vi "ReadFFLoop.vi"(0 "blocktrigger":u8, 1 "btrig_ch":u8, 2 "ExtTrig":u8, 3 "cam_sel":u8, 4 "freq":u32, 5 "exptus":u32=20000) -> ()   [LabVIEW 2015]
uses:
  ESLSCDLL.dll
panel:
  # "lines for  FFTs, or 0 else"
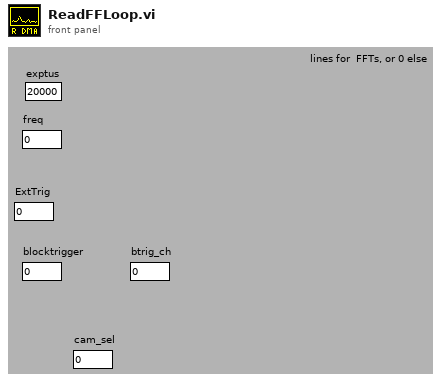
[diagram p1: front panel]
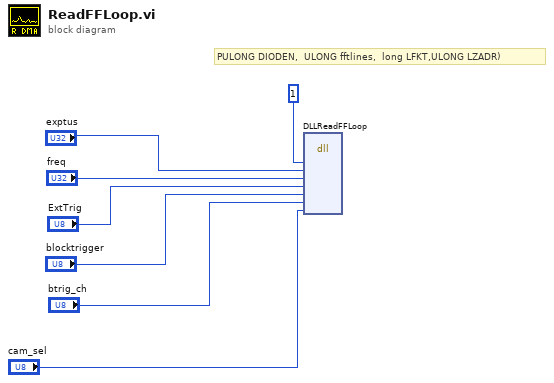
[diagram p0: block diagram]
diagram:
  # "PULONG DIODEN, \tULONG fftlines,  long LFKT,ULONG LZADR)"
  n1 = dll-call lib="C:/ENTW/PCIE/64bit/lv64/2camx/board.vis/ESLSCDLL.dll" fn="DLLReadFFLoop"("drv"=u32 1, "exptus"="exptus", "freq"="freq", "exttrig"="ExtTrig", "blocktrigger"="blocktrigger", "btrig_ch"="btrig_ch", "cam_sel"="cam_sel") -> ()  [unwired: 11 in, 2 out]
